vi "get_ref.vi"(8 "error in (no error)":errorcluster, 9 "Name":string="Trigger", 11 "VI reference":refnum<vi>) -> (0 "error out":errorcluster, 1 "Controls":string[](array[string]), 2 "Ctrl reference out":refnum<vi>, 3 "VI reference out":refnum<vi>)   [LabVIEW 2015, in "oskar_tools.lvlib"]
uses:
  oskar_tools.lvlib
panel:
  out "Controls":i32
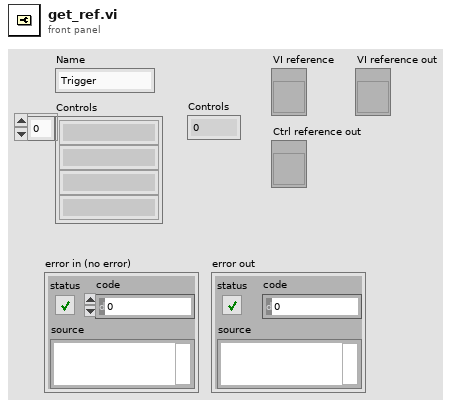
[diagram p1: front panel]
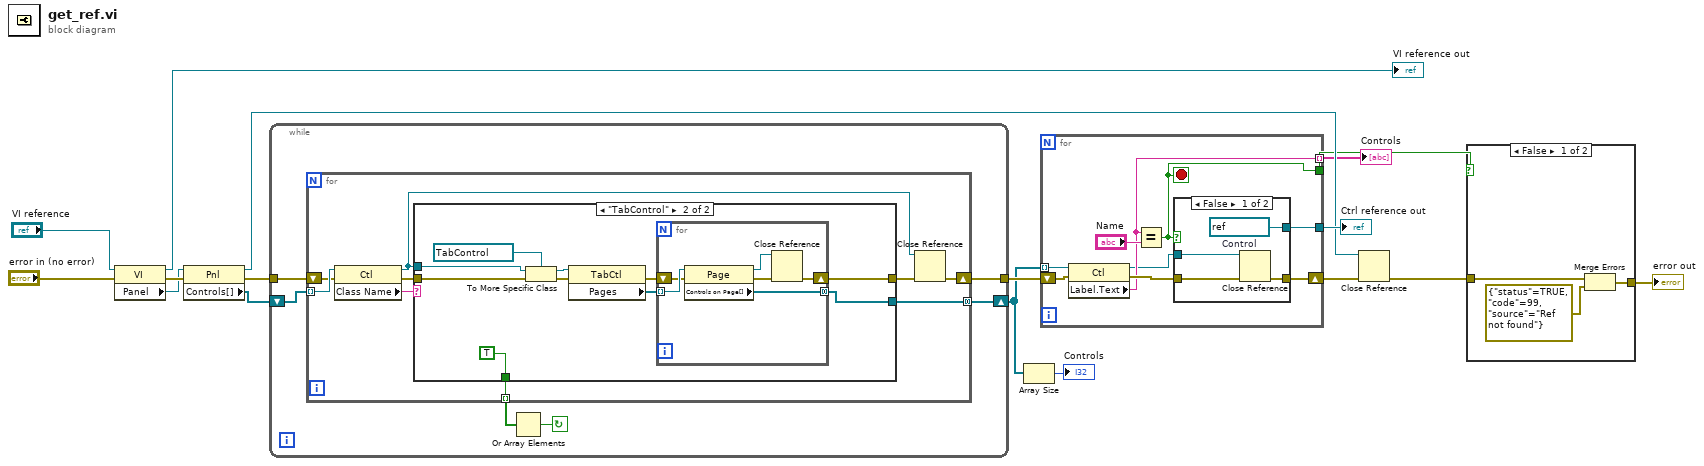
[diagram p0: block diagram]
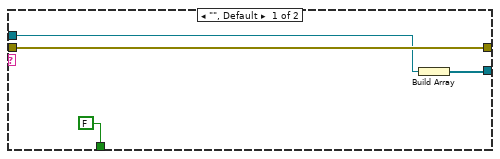
[diagram p2: hidden frame]
diagram:
  n1 = property class="VI"(reference="VI reference", error in="error in (no error)") -> (reference out=→"VI reference out":refnum<vi>, error out=w17:errorcluster, "Panel"=w16:refnum<vi>)
  n2 = property class="Pnl"(reference=w16, error in=w17) -> (reference out=w9:refnum<vi>, error out=w14:errorcluster, "Controls[]"=w4:refnum<vi>[])
  n3 = while {
    tunnel: w14 -> [w23]
    tunnel: [w22] -> w13
    shift-right: [w18] -> w2
    shift-left: w4 -> [w21]
    stop <- w19 continue-if-true
    n4 = for {
      tunnel: w21 -> [w29] mode=indexing
      shift-right: [w32] -> w22
      shift-left: w23 -> [w28]
      tunnel: [w25] -> w20 mode=indexing
      tunnel: [w24] -> w18 mode=concatenating
      n5 = property class="Ctl"(reference=w29, error in=w28) -> (reference out=w27:refnum<vi>, error out=w31:errorcluster, "Class Name"=w26:string)
      n6 = case shown="\"TabControl\"" w26 {
        tunnel: w27 -> [w33 w43]
        tunnel: w31 -> [w36 w41]
        tunnel: [w36 w39] -> w30
        tunnel: [w34 w37] -> w24
        tunnel: [FALSE TRUE] -> w25
        frame "", Default {
          n7 = Build Array(w33) -> (w34:refnum<vi>[])
        }
        frame "TabControl" {
          n8 = To More Specific Class(target class=refnum<vi> refnum ("Tab Control"), reference=w43, error in=w41) -> (specific class reference=w46:refnum<vi>, error out=w45:errorcluster)
          n9 = property class="TabCtl"(reference=w46, error in=w45) -> (error out=w40:errorcluster, "Pages"=w42:refnum<vi>[])  [unwired: 1 out]
          n10 = for {
            tunnel: w42 -> [w52] mode=indexing
            shift-right: [w49] -> w39
            shift-left: w40 -> [w51]
            tunnel: [w48] -> w37 mode=concatenating
            n11 = property class="Page"(reference=w52, error in=w51) -> (reference out=w50:refnum<vi>, error out=w47:errorcluster, "Controls on Page[]"=w48:refnum<vi>[])
            n12 = Close Reference(reference=w50, error in (no error)=w47) -> (error out=w49:errorcluster)
          }
        }
      }
      n13 = Close Reference(reference=w27, error in (no error)=w30) -> (error out=w32:errorcluster)
    }
    n14 = Or Array Elements(Boolean array=w20) -> (logical OR=w19:bool)
  }
  n15 = Array Size(array=w2) -> (size(s)=→"Controls":i32)
  n16 = for {
    tunnel: w2 -> [w59] mode=indexing
    tunnel: [w54] -> w12
    shift-right: [w57] -> w10
    shift-left: w13 -> [w60]
    tunnel: [w56] -> w8 mode=indexing
    tunnel: [w53] -> w6
    stop <- w53 stop-if-true
    n17 = property class="Ctl"(reference=w59, error in=w60) -> (reference out=w55:refnum<vi>, error out=w58:errorcluster, "Label.Text"=w56:string)
    n18 = Equal?(x=w56, y="Name") -> (x = y?=w53:bool)
    n19 = case shown="False" w53 {
      tunnel: w58 -> [w65 w67]
      tunnel: [w64 w67] -> w57
      tunnel: w55 -> [w63 w66]
      tunnel: [w62 w66] -> w54
      frame False {
        w62 = refnum<vi> refnum  # Control
        n20 = Close Reference(reference=w63, error in (no error)=w65) -> (error out=w64:errorcluster)
      }
      frame True {
      }
    }
  }
  "Ctrl reference out" <- w12
  "Controls" <- w8
  n21 = Close Reference(reference=w9, error in (no error)=w10) -> (error out=w3:errorcluster)
  n22 = case shown="False" w6 {
    tunnel: w3 -> [w69 w71]
    tunnel: [w68 w71] -> w7
    frame False {
      n23 = Merge Errors(w69, errorcluster {"status"=TRUE, "code"=99, "source"="Ref not found"} ("error in (no error)")) -> (w68:errorcluster)
    }
    frame True {
    }
  }
  "error out" <- w7
